vi "user action.vi"(8 "error in":errorcluster, 9 "Cash":string="Cash", 10 "Users data":T2, 11 "user action":T4) -> (0 "error out":errorcluster, 1 "Messageout":T1, 2 "Output":string, 3 "Users data out":T2)   [LabVIEW 2015]
uses:
  Controls/Users data.ctl
  Controls/user.ctl
  Controls/useraction.ctl
  Controls/message.ctl
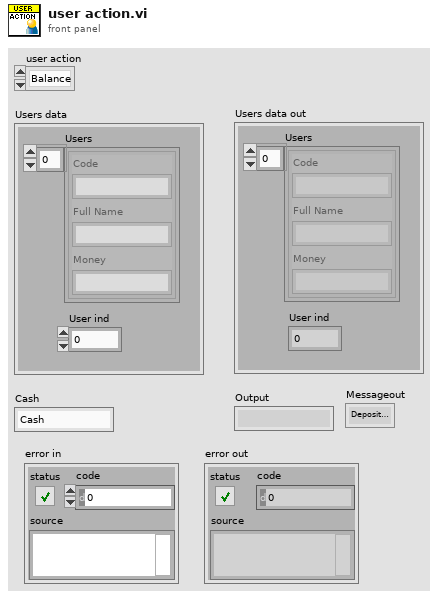
[diagram p1: front panel]
types:
  T1 = typedef "message.ctl" = enum16{"Deposit Complete", "Welcome", "Menu", "Verification Failed", "Session Terminate", "Deposit", "Withdrawal", "Withdrawal Complete", "Withdrawal Failed", "Balance Inq"}
  T2 = typedef "Users data.ctl" = cluster{"Users ":T3[], "User ind":i32}
  T3 = typedef "user.ctl" = cluster{"Full Name":string, "Code":string, "Money":string}
  T4 = typedef "useraction.ctl" = enum16{"Balance", "Withdraw", "Deposit"}
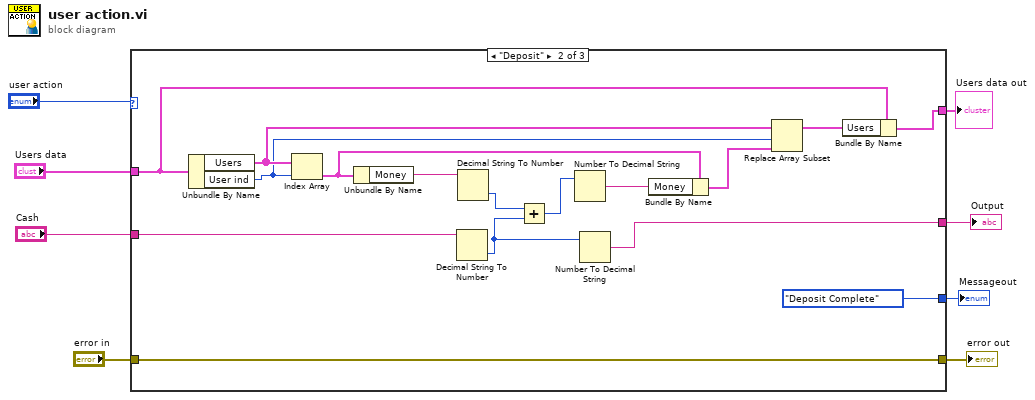
[diagram p0: block diagram]
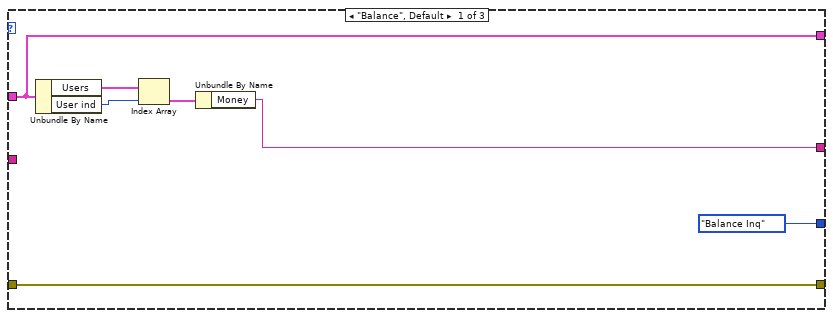
[diagram p2: hidden frame]
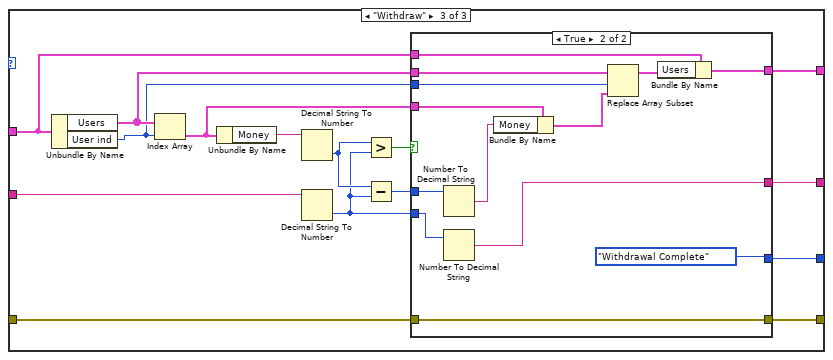
[diagram p3: hidden frame]
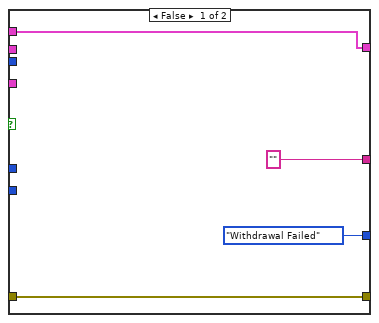
[diagram p4: hidden frame]
diagram:
  n1 = case shown="\"Deposit\"" "user action" {
    tunnel: "Users data" -> [w11 w22 w36]
    tunnel: "Cash" -> [_ w30 w45]
    tunnel: [w12 w16 w39] -> w7
    tunnel: [w11 w20 w35] -> w8
    tunnel: "error in" -> [w10 w19 w34]
    tunnel: [w10 w19 w33] -> w2
    tunnel: [message."Balance Inq" ("Message in") message."Deposit Complete" ("Message in") w32] -> w1
    frame "Balance", Default {
      n2 = Unbundle By Name(w11) -> ("Users"=w15:T3[], "User ind"=w14:i32)
      n3 = Index Array(array=w15, index=w14) -> (element=w13:T3)
      n4 = Unbundle By Name(w13) -> ("Money"=w12:string)
    }
    frame "Deposit" {
      n5 = Unbundle By Name(w22) -> ("Users"=w26:T3[], "User ind"=w25:i32)
      n6 = Index Array(array=w26, index=w25) -> (element=w27:T3)
      n7 = Unbundle By Name(w27) -> ("Money"=w31:string)
      n8 = Decimal String To Number(string=w30) -> (number=w17:i32)  [unwired: 2 in, 1 out]
      n9 = Decimal String To Number(string=w31) -> (number=w29:i32)  [unwired: 2 in, 1 out]
      n10 = Add(x=w29, y=w17) -> (x+y=w28:i32)
      n11 = Number To Decimal String(number=w28) -> (decimal integer string=w23:string)  [unwired: 1 in]
      n12 = Number To Decimal String(number=w17) -> (decimal integer string=w16:string)  [unwired: 1 in]
      n13 = Bundle By Name(cluster=w27, "Money"=w23) -> (w24:T3)
      n14 = Replace Array Subset(array=w26, new element=w24, index=w25) -> (w21:T3[])
      n15 = Bundle By Name(cluster=w22, "Users"=w21) -> (w20:T2)
    }
    frame "Withdraw" {
      n16 = Unbundle By Name(w36) -> ("Users"=w38:T3[], "User ind"=w37:i32)
      n17 = Index Array(array=w38, index=w37) -> (element=w43:T3)
      n18 = Unbundle By Name(w43) -> ("Money"=w46:string)
      n19 = Decimal String To Number(string=w46) -> (number=w42:i32)  [unwired: 2 in, 1 out]
      n20 = Decimal String To Number(string=w45) -> (number=w40:i32)  [unwired: 2 in, 1 out]
      n21 = Greater?(x=w42, y=w40) -> (0:w44:bool)
      n22 = Subtract(x=w42, y=w40) -> (x-y=w41:i32)
      n23 = case shown="True" w44 {
        tunnel: w43 -> [_ w62]
        tunnel: w41 -> [_ w63]
        tunnel: w40 -> [_ w60]
        tunnel: ["" w59] -> w39
        tunnel: w38 -> [_ w58]
        tunnel: w37 -> [_ w56]
        tunnel: w36 -> [w48 w55]
        tunnel: [w48 w53] -> w35
        tunnel: w34 -> [w49 w52]
        tunnel: [w49 w52] -> w33
        tunnel: [message."Withdrawal Failed" ("Message in") message."Withdrawal Complete" ("Message in")] -> w32
        frame False {
        }
        frame True {
          n24 = Number To Decimal String(number=w63) -> (decimal integer string=w61:string)  [unwired: 1 in]
          n25 = Number To Decimal String(number=w60) -> (decimal integer string=w59:string)  [unwired: 1 in]
          n26 = Bundle By Name(cluster=w62, "Money"=w61) -> (w57:T3)
          n27 = Replace Array Subset(array=w58, new element=w57, index=w56) -> (w54:T3[])
          n28 = Bundle By Name(cluster=w55, "Users"=w54) -> (w53:T2)
        }
      }
    }
  }
  "Output" <- w7
  "Users data out" <- w8
  "error out" <- w2
  "Messageout" <- w1
